vi "setsnjob.vi"(3 "sample sn":string[](array[string]), 4 "sample old sn":string[](array[string]), 5 "sample port":refnum<visa-resource-name>[](array[refnum])) -> (0 "sample sn out":string[](array[string]))   [LabVIEW 2012]
uses:
  globalstatus.vi
  globalreport.vi
panel:
  out "error":errorcluster[](array[cluster])
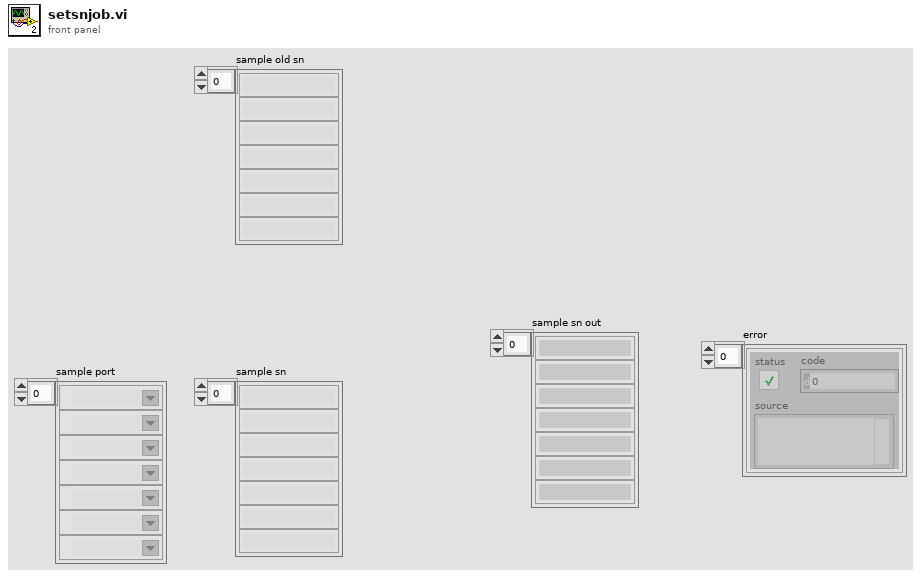
[diagram p1: front panel]
types:
  T1 = cluster{"PORT":string, "SN":string, "RED DAC":dbl, "BLUE DAC":dbl, "RED AMP":dbl, "BLUE AMP":dbl, "T0":dbl, "T1":dbl, "T2":dbl, "T3":dbl, "T4":dbl, "T5":dbl, "T6":dbl, "A0":dbl, "A1":dbl, "A2":dbl, "A3":dbl, "B0":dbl, "B1":dbl, "B2":dbl, "C1":dbl, "C0":dbl, "result":string, "error":string}[]
  T2 = cluster{"PORT":string, "sample sn":string, "RED DAC":dbl, "BLUE DAC":dbl, "RED AMP":dbl, "BLUE AMP":dbl, "T0":dbl, "T1":dbl, "T2":dbl, "T3":dbl, "T4":dbl, "T5":dbl, "T6":dbl, "A0":dbl, "A1":dbl, "A2":dbl, "A3":dbl, "B0":dbl, "B1":dbl, "B2":dbl, "C1":dbl, "C0":dbl, string, string}
  T3 = cluster{"PORT":string, "sample sn":string, "RED DAC":dbl, "BLUE DAC":dbl, "RED AMP":dbl, "BLUE AMP":dbl, "T0":dbl, "T1":dbl, "T2":dbl, "T3":dbl, "T4":dbl, "T5":dbl, "T6":dbl, "A0":dbl, "A1":dbl, "A2":dbl, "A3":dbl, "B0":dbl, "B1":dbl, "B2":dbl, "C1":dbl, "C0":dbl, "result":string, "error":string}
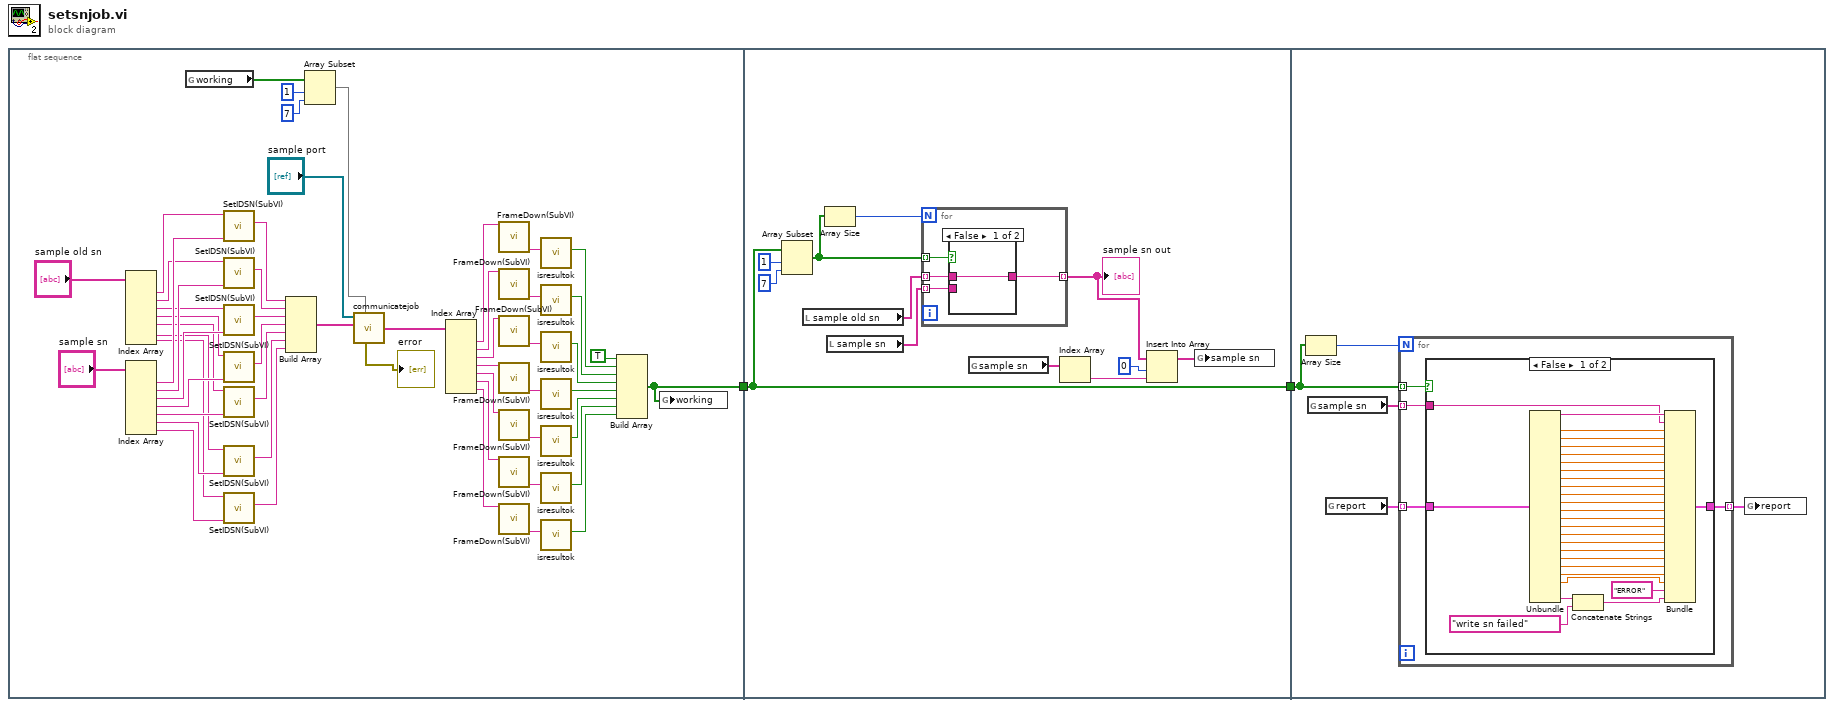
[diagram p0: block diagram]
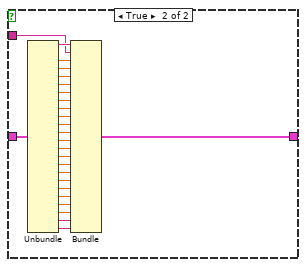
[diagram p3: hidden frame]
diagram:
  n1 = flat-sequence {
    tunnel: [w3] -> w2
    tunnel: w2 -> [w57]
    tunnel: [w57] -> w1
    tunnel: w1 -> [w75]
    frame #0 {
      n2 = Index Array(array="sample old sn") -> (element #1=w15:string, element #2=w14:string, element #3=w13:string, element #4=w12:string, element #5=w11:string, element #6=w10:string, element #7=w9:string)  [unwired: 7 in]
      n3 = Index Array(array="sample sn") -> (element #1=w56:string, element #2=w55:string, element #3=w54:string, element #4=w53:string, element #5=w52:string, element #6=w51:string, element #7=w50:string)  [unwired: 7 in]
      n4 = global read "globalstatus.vi" "working"() -> (w7:bool[])
      n5 = call "SetIDSN(SubVI).vi"("input sn"=w56, "sn"=w15) -> ("output frame"=w47:string)  [unwired: 9 in]
      n6 = call "SetIDSN(SubVI).vi"("input sn"=w55, "sn"=w14) -> ("output frame"=w46:string)  [unwired: 9 in]
      n7 = call "SetIDSN(SubVI).vi"("input sn"=w54, "sn"=w13) -> ("output frame"=w45:string)  [unwired: 9 in]
      n8 = call "SetIDSN(SubVI).vi"("input sn"=w53, "sn"=w12) -> ("output frame"=w44:string)  [unwired: 9 in]
      n9 = call "SetIDSN(SubVI).vi"("input sn"=w52, "sn"=w11) -> ("output frame"=w43:string)  [unwired: 9 in]
      n10 = call "SetIDSN(SubVI).vi"("input sn"=w51, "sn"=w10) -> ("output frame"=w42:string)  [unwired: 9 in]
      n11 = call "SetIDSN(SubVI).vi"("input sn"=w50, "sn"=w9) -> ("output frame"=w41:string)  [unwired: 9 in]
      n12 = Build Array(w47, w46, w45, w44, w43, w42, w41) -> (w40:string[])
      n13 = Array Subset(array=w7, index=1, length=7) -> (w6:bool[])
      n14 = call "communicatejob.vi"("sample port"="sample port", "condition"=w6, "send command"=w40) -> ("error"=→"error":errorcluster[], "receive command"=w24:string[])  [unwired: 2 in, 2 out]
      n15 = Index Array(array=w24) -> (element #1=w23:string, element #2=w22:string, element #3=w21:string, element #4=w20:string, element #5=w19:string, element #6=w18:string, element #7=w17:string)  [unwired: 7 in]
      n16 = call "FrameDown(SubVI).vi"("input frame"=w23) -> ("result"=w38:string)  [unwired: 4 in, 10 out]
      n17 = call "FrameDown(SubVI).vi"("input frame"=w22) -> ("result"=w33:string)  [unwired: 4 in, 10 out]
      n18 = call "FrameDown(SubVI).vi"("input frame"=w21) -> ("result"=w36:string)  [unwired: 4 in, 10 out]
      n19 = call "FrameDown(SubVI).vi"("input frame"=w20) -> ("result"=w39:string)  [unwired: 4 in, 10 out]
      n20 = call "FrameDown(SubVI).vi"("input frame"=w19) -> ("result"=w34:string)  [unwired: 4 in, 10 out]
      n21 = call "FrameDown(SubVI).vi"("input frame"=w18) -> ("result"=w37:string)  [unwired: 4 in, 10 out]
      n22 = call "FrameDown(SubVI).vi"("input frame"=w17) -> ("result"=w35:string)  [unwired: 4 in, 10 out]
      n23 = call "isresultok.vi"("result"=w38) -> ("ok"=w26:bool)  [unwired: 10 in]
      n24 = call "isresultok.vi"("result"=w33) -> ("ok"=w27:bool)  [unwired: 10 in]
      n25 = call "isresultok.vi"("result"=w36) -> ("ok"=w28:bool)  [unwired: 10 in]
      n26 = call "isresultok.vi"("result"=w39) -> ("ok"=w29:bool)  [unwired: 10 in]
      n27 = call "isresultok.vi"("result"=w34) -> ("ok"=w30:bool)  [unwired: 10 in]
      n28 = call "isresultok.vi"("result"=w37) -> ("ok"=w31:bool)  [unwired: 10 in]
      n29 = call "isresultok.vi"("result"=w35) -> ("ok"=w32:bool)  [unwired: 10 in]
      n30 = Build Array(TRUE, w26, w27, w28, w29, w30, w31, w32) -> (w3:bool[])
      n31 = global write "globalstatus.vi" "working"(w3) -> ()
    }
    frame #1 {
      n32 = Array Subset(array=w57, index=1, length=7) -> (w60:bool[])
      n33 = local read "sample old sn"() -> (w66:string[])
      n34 = Array Size(array=w60) -> (size(s)=w68:i32)
      n35 = local read "sample sn"() -> (w67:string[])
      n36 = for {
        N: w68 -> [_]
        tunnel: w60 -> [w72] mode=indexing
        tunnel: w67 -> [w71] mode=indexing
        tunnel: [w70] -> w61 mode=indexing
        tunnel: w66 -> [w69] mode=indexing
        n37 = case shown="False" w72 {
          tunnel: w71 -> [_ w74]
          tunnel: [w73 w74] -> w70
          tunnel: w69 -> [w73 _]
          frame False {
          }
          frame True {
          }
        }
      }
      "sample sn out" <- w61
      n38 = global read "globalstatus.vi" "sample sn"() -> (w64:string[])
      n39 = Index Array(array=w64) -> (element=w63:string)  [unwired: 1 in]
      n40 = Insert Into Array(array=w61, index=0, new element=w63) -> (w62:string[])
      n41 = global write "globalstatus.vi" "sample sn"(w62) -> ()
    }
    frame #2 {
      n42 = Array Size(array=w75) -> (size(s)=w79:i32)
      n43 = global read "globalstatus.vi" "sample sn"() -> (w76:string[])
      n44 = global read "globalreport.vi" "report"() -> (w77:T1)
      n45 = for {
        N: w79 -> [_]
        tunnel: w77 -> [w83] mode=indexing
        tunnel: [w82] -> w78 mode=indexing
        tunnel: w75 -> [w81] mode=indexing
        tunnel: w76 -> [w80] mode=indexing
        n46 = case shown="False" w81 {
          tunnel: w83 -> [w89 w137]
          tunnel: w80 -> [w84 w112]
          tunnel: [w90 w113] -> w82
          frame False {
            n47 = Unbundle(w89) -> ("PORT"=w111:string, "RED DAC"=w110:dbl, "BLUE DAC"=w109:dbl, "RED AMP"=w108:dbl, "BLUE AMP"=w107:dbl, "T0"=w106:dbl, "T1"=w105:dbl, "T2"=w104:dbl, "T3"=w103:dbl, "T4"=w102:dbl, "T5"=w101:dbl, "T6"=w100:dbl, "A0"=w99:dbl, "A1"=w98:dbl, "A2"=w97:dbl, "A3"=w96:dbl, "B0"=w95:dbl, "B1"=w94:dbl, "B2"=w93:dbl, "C1"=w92:dbl, "C0"=w91:dbl, "error"=w87:string)  [unwired: 2 out]
            n48 = Concatenate Strings(w87, "write sn failed") -> (w85:string)
            n49 = Bundle("PORT"=w111, "sample sn"=w84, "RED DAC"=w110, "BLUE DAC"=w109, "RED AMP"=w108, "BLUE AMP"=w107, "T0"=w106, "T1"=w105, "T2"=w104, "T3"=w103, "T4"=w102, "T5"=w101, "T6"=w100, "A0"=w99, "A1"=w98, "A2"=w97, "A3"=w96, "B0"=w95, "B1"=w94, "B2"=w93, "C1"=w92, "C0"=w91, "ERROR", w85) -> (w90:T2)  [unwired: 1 in]
          }
          frame True {
            n50 = Unbundle(w137) -> ("PORT"=w136:string, "RED DAC"=w135:dbl, "BLUE DAC"=w134:dbl, "RED AMP"=w133:dbl, "BLUE AMP"=w132:dbl, "T0"=w131:dbl, "T1"=w130:dbl, "T2"=w129:dbl, "T3"=w128:dbl, "T4"=w127:dbl, "T5"=w126:dbl, "T6"=w125:dbl, "A0"=w124:dbl, "A1"=w123:dbl, "A2"=w122:dbl, "A3"=w121:dbl, "B0"=w120:dbl, "B1"=w119:dbl, "B2"=w118:dbl, "C1"=w117:dbl, "C0"=w116:dbl, "result"=w115:string, "error"=w114:string)  [unwired: 1 out]
            n51 = Bundle("PORT"=w136, "sample sn"=w112, "RED DAC"=w135, "BLUE DAC"=w134, "RED AMP"=w133, "BLUE AMP"=w132, "T0"=w131, "T1"=w130, "T2"=w129, "T3"=w128, "T4"=w127, "T5"=w126, "T6"=w125, "A0"=w124, "A1"=w123, "A2"=w122, "A3"=w121, "B0"=w120, "B1"=w119, "B2"=w118, "C1"=w117, "C0"=w116, "result"=w115, "error"=w114) -> (w113:T3)  [unwired: 1 in]
          }
        }
      }
      n52 = global write "globalreport.vi" "report"(w78) -> ()
    }
  }
